vi "Variant2Integer.vi"(8 "error in (no error)":errorcluster, 11 "Variant":variant) -> (0 "error out":errorcluster, 3 "data":i32)   [LabVIEW 2020]
uses:
  <vilib>/Utility/Data Type/Type Definitions/Data Type.ctl
  <vilib>/Utility/Data Type/NI_Data Type.lvlib
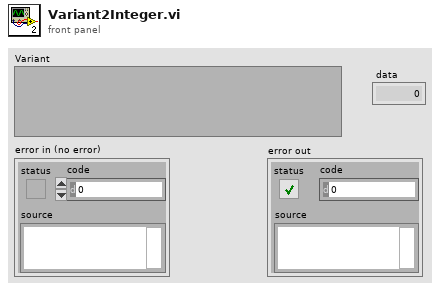
[diagram p1: front panel]
types:
  T1 = typedef "NI_Data Type.lvlib/Data Type.ctl" = enum8{"Invalid Type", "Void", "I8", "I16", "I32", "I64", "U8", "U16", "U32", "U64", "Single Float", "Double Float", "Extended Float", "Single Complex", "Double Complex", "Extended Complex", "Enum U8", "Enum U16", "Enum U32", "Enum U64", "Single Float With Unit", "Double Float With Unit", "Extended Float With Unit", "Single Complex with Unit", "Double Complex with Unit", "Extended Complex with Unit", "Boolean", "String", "Path", "Picture", "Tag", "Array", "Cluster", "Variant", "LV Variant", "Waveform", "Timestamp", "Digital Waveform", "Digital Data", "ExpressData", "Refnum", "External Data", "VI", "Poly VI", "LabVIEW Class Instance", "Fixed Point", "Set Collection", "Map Collection"}
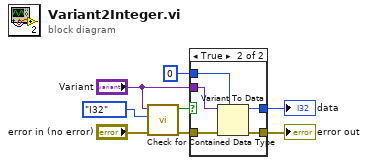
[diagram p0: block diagram]
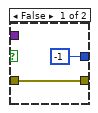
[diagram p2: hidden frame]
diagram:
  n1 = call <vilib>:"Check for Contained Data Type.vi"("error in (no error)"="error in (no error)", "data type to find"=Data_Type."I32" ("Data Type to Find"), "variant"="Variant") -> ("error out"=w4:errorcluster, "contains data type to find?"=w6:bool)  [unwired: 7 in]
  n2 = case shown="True" w6 {
    tunnel: [-1 w15] -> w8
    tunnel: "Variant" -> [_ w14]
    tunnel: 0 -> [_ w13]
    tunnel: w4 -> [w9 w12]
    tunnel: [w9 w11] -> w2
    frame False {
    }
    frame True {
      n3 = Variant To Data(error in=w12, type=w13, Variant=w14) -> (data=w15:i32, error out=w11:errorcluster)
    }
  }
  "data" <- w8
  "error out" <- w2
